vi "2017-03-23 TTTR Test.vi"() -> ()   [LabVIEW 2016]
uses:
  Program Files/PicoQuant/HydraHarp-HHLibv30/demos/64bit/LabVIEW/LabView2013/ttrmode.llb/Global.vi
  HHLib64.dll
panel:
  in  "Acq.Time":i32=10000 min=1 max=3600000 step=100
  out "FiFo Overrun":bool
  out "OK":bool
  out "Counts":i32
  in  "Path":path=path "C:/Users/WilsonLab1/Desktop/test"
  out "Initialization Status":string
  out "Serial":string
  out "DLL Version":string
  out "DevIdx":dbl
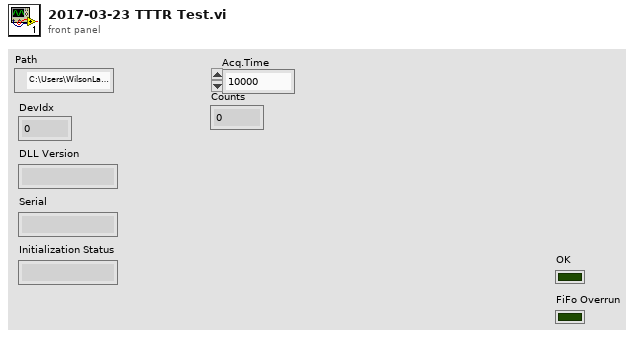
[diagram p1: front panel]
types:
  T1 = enum16{"open", "replace", "create", "open or create", "replace or create", "replace or create with confirmation"}
  T2 = cluster{"rate":i32, "rate":i32, "rate":i32, "rate":i32, "rate":i32, "rate":i32, "rate":i32, "rate":i32}
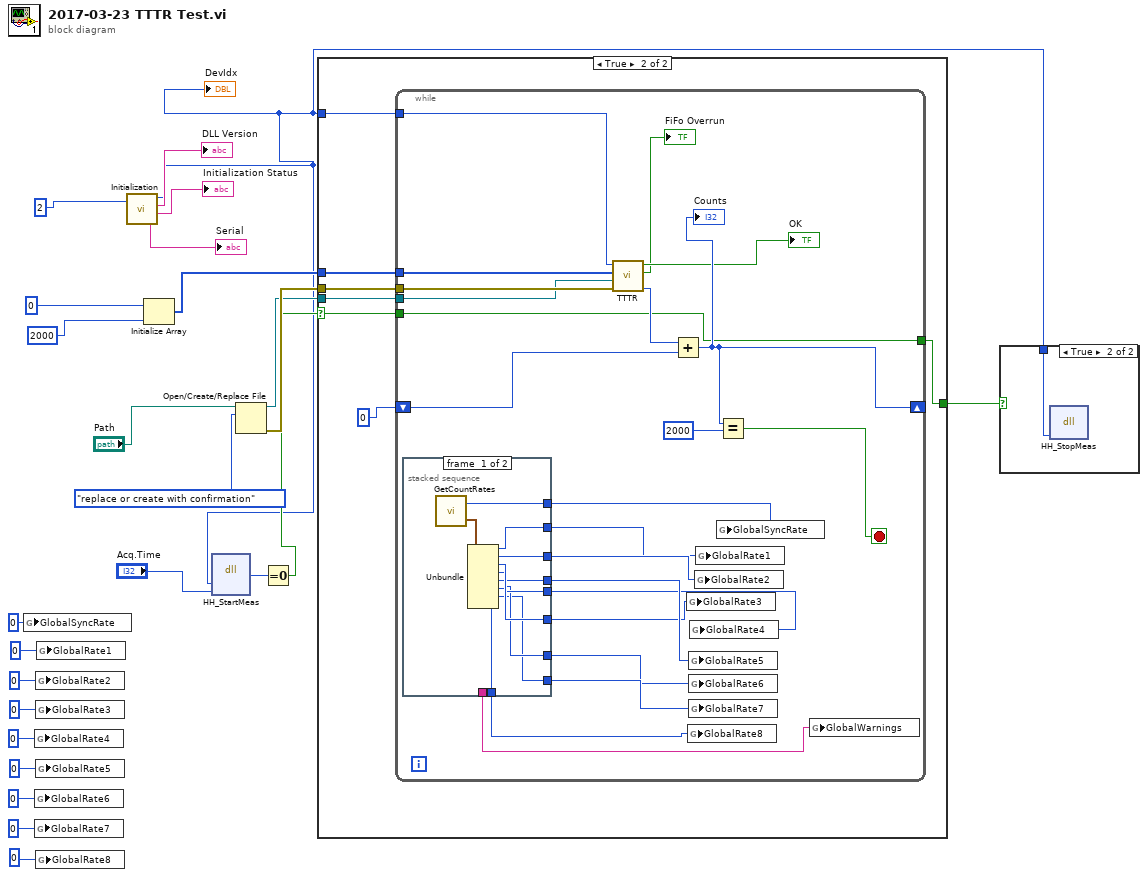
[diagram p0: block diagram]
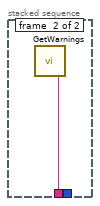
[diagram p4: hidden frame]
diagram:
  n1 = global write "Global.vi" "GlobalSyncRate"(0) -> ()
  n2 = global write "Global.vi" "GlobalRate4"(0) -> ()
  n3 = global write "Global.vi" "GlobalRate6"(0 ("GlobalRate6")) -> ()
  n4 = global write "Global.vi" "GlobalRate7"(0 ("GlobalRate7")) -> ()
  n5 = global write "Global.vi" "GlobalRate2"(0) -> ()
  n6 = global write "Global.vi" "GlobalRate3"(0) -> ()
  n7 = global write "Global.vi" "GlobalRate5"(0 ("GlobalRate5")) -> ()
  n8 = global write "Global.vi" "GlobalRate8"(0 ("GlobalRate8")) -> ()
  n9 = global write "Global.vi" "GlobalRate1"(0) -> ()
  n10 = call "Initialization.vi"("Mode"=2) -> ("Deviceindex"=w1:i32, "DLL Version"=→"DLL Version":string, "Initialization Status"=→"Initialization Status":string, "Serial[8]"=→"Serial":string)  [unwired: 1 out]
  "DevIdx" <- w1
  n11 = Initialize Array(0, 2000) -> (w15:i32[])
  n12 = dll-call lib="hhlib64.dll" fn="HH_StartMeas"("devidx"=w1, "tacq"="Acq.Time") -> ("return type"=w5:i32)  [unwired: 5 in, 2 out]
  n13 = Open/Create/Replace File(file path (use dialog)="Path", operation (0:open)=T1."replace or create with confirmation") -> (refnum out=w16:refnum<file>, error out=w17:errorcluster)  [unwired: 4 in, 1 out]
  n14 = Equal To 0?(x=w5) -> (x = 0?=w3:bool)
  n15 = case shown="True" w3 {
    selector: w3 -> [w26 w29]
    tunnel: w17 -> [_ w33]
    tunnel: w16 -> [_ w32]
    tunnel: w15 -> [_ w31]
    tunnel: w1 -> [_ w30]
    tunnel: [w26 w28] -> w2
    frame False {
    }
    frame True {
      n16 = while {
        tunnel: w33 -> [w55]
        shift-right: [w50] -> _
        shift-left: 0 -> [w54]
        tunnel: w32 -> [w47]
        tunnel: w31 -> [w46]
        tunnel: w30 -> [w45]
        tunnel: [w34] -> w28
        tunnel: w29 -> [w34]
        stop <- w51 stop-if-true
        n17 = stacked-sequence {
          tunnel: [w64 _] -> w35
          tunnel: [w63 _] -> w36
          tunnel: [w62 _] -> w37
          tunnel: [w61 _] -> w38
          tunnel: [w60 _] -> w39
          tunnel: [w59 _] -> w40
          tunnel: [w58 _] -> w41
          tunnel: [w57 _] -> w42
          tunnel: [w56 _] -> w43
          tunnel: [_ w66] -> w44
          frame #0 {
            n18 = call "GetCountRates.vi"() -> ("SyncRate"=w64:i32, "Count Rates"=w65:T2)  [unwired: 1 in]
            n19 = Unbundle(w65) -> ("rate"=w63:i32, "rate"=w62:i32, "rate"=w61:i32, "rate"=w60:i32, "rate"=w59:i32, "rate"=w58:i32, "rate"=w57:i32, "rate"=w56:i32)
          }
          frame #1 {
            n20 = call "GetWarnings.vi"() -> ("warningstext"=w66:string)  [unwired: 1 in]
          }
        }
        n21 = call "TTTR.vi"("error in (no error)"=w55, "file refnum"=w47, "Array"=w46, "DeviceIndex"=w45) -> ("count"=w53:i32, "FiFoOverrun"=→"FiFo Overrun":bool, "OK"=→"OK":bool)  [unwired: 1 out]
        n22 = Add(x=w53, y=w54) -> (x+y=w50:i32)
        "Counts" <- w50
        n23 = global write "Global.vi" "GlobalRate3"(w38) -> ()
        n24 = global write "Global.vi" "GlobalRate8"(w43) -> ()
        n25 = global write "Global.vi" "GlobalRate5"(w40) -> ()
        n26 = global write "Global.vi" "GlobalRate6"(w41) -> ()
        n27 = global write "Global.vi" "GlobalRate7"(w42) -> ()
        n28 = global write "Global.vi" "GlobalRate4"(w39) -> ()
        n29 = global write "Global.vi" "GlobalRate2"(w37) -> ()
        n30 = global write "Global.vi" "GlobalRate1"(w36) -> ()
        n31 = global write "Global.vi" "GlobalSyncRate"(w35) -> ()
        n32 = Equal?(x=w50, y=2000) -> (x = y?=w51:bool)
        n33 = global write "Global.vi" "GlobalWarnings"(w44) -> ()
      }
    }
  }
  n34 = case shown="True" w2 {
    tunnel: w1 -> [_ w67]
    frame False {
    }
    frame True {
      n35 = dll-call lib="hhlib64.dll" fn="HH_StopMeas"("devidx"=w67) -> ()  [unwired: 5 in, 2 out]
    }
  }
